vi "Setmode.vi"(8 "error in (no error)":errorcluster, 10 "Set_Val":T1, 11 "OneOfTemplate in":refnum<class "nixnet_grpc_CreateSessionByRefRequest_mode_enum.lvclass">) -> (0 "error out":errorcluster, 3 "OneOfTemplate out":refnum<class "nixnet_grpc_CreateSessionByRefRequest_mode_enum.lvclass">)   [LabVIEW 2019, in "xnet-grpc_client.lvlib" / "nixnet_grpc_CreateSessionByRefRequest_mode_enum.lvclass"]
uses:
  nixnet_grpc_CreateSessionByRefRequest_mode_enum.lvclass
  nixnet_grpc_CreateSessionMode.ctl
  nixnet_grpc_CreateSessionByRefRequest_mode_enum.lvclass/nixnet_grpc_CreateSessionByRefRequest_mode_enum.ctl
  xnet-grpc_client.lvlib
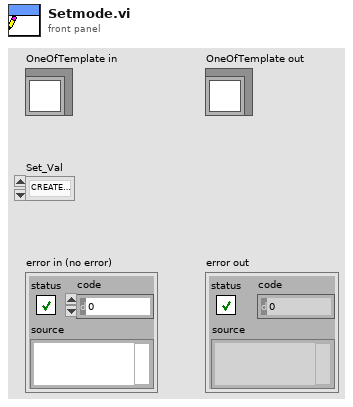
[diagram p1: front panel]
types:
  T1 = typedef "xnet-grpc_client.lvlib/nixnet_grpc_CreateSessionMode.ctl" = enum32{"CREATE_SESSION_MODE_SIGNAL_IN_SINGLE_POINT", "CREATE_SESSION_MODE_SIGNAL_IN_WAVEFORM", "CREATE_SESSION_MODE_SIGNAL_IN_XY", "CREATE_SESSION_MODE_SIGNAL_OUT_SINGLE_POINT", "CREATE_SESSION_MODE_SIGNAL_OUT_WAVEFORM", "CREATE_SESSION_MODE_SIGNAL_OUT_XY", "CREATE_SESSION_MODE_FRAME_IN_STREAM", "CREATE_SESSION_MODE_FRAME_IN_QUEUED", "CREATE_SESSION_MODE_FRAME_IN_SINGLE_POINT", "CREATE_SESSION_MODE_FRAME_OUT_STREAM", "CREATE_SESSION_MODE_FRAME_OUT_QUEUED", "CREATE_SESSION_MODE_FRAME_OUT_SINGLE_POINT", "CREATE_SESSION_MODE_SIGNAL_CONVERSION_SINGLE_POINT"}
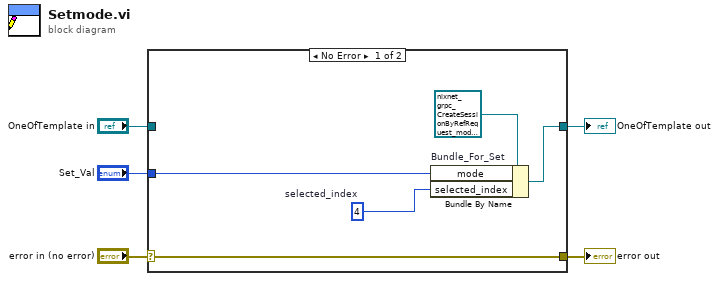
[diagram p0: block diagram]
diagram:
  n1 = case shown="No Error" "error in (no error)" {
    selector: "error in (no error)" -> [w10 w11]
    tunnel: [w10 w11] -> w4
    tunnel: [w9 w12] -> w2
    tunnel: "OneOfTemplate in" -> [_ w12]
    tunnel: "Set_Val" -> [w8 _]
    frame No Error {
      w7 = 4  # selected_index
      n2 = Bundle By Name "Bundle_For_Set"(cluster=refnum<class "nixnet_grpc_CreateSessionByRefRequest_mode_enum.lvclass"> refnum ("OneOfTemplate in"), "mode"=w8, "selected_index"=w7) -> (w9:refnum<class "nixnet_grpc_CreateSessionByRefRequest_mode_enum.lvclass">)
    }
    frame Error {
    }
  }
  "error out" <- w4
  "OneOfTemplate out" <- w2
